vi "Dirac Integrand for Gated Decay.vi"(8 "Error In":errorcluster, 11 "data":variant) -> (0 "Error Out":errorcluster, 3 "F(X)":dbl)   [LabVIEW 2021, in "Phasor.lvlib"]
doc: "This template is the starting point for creating a function that is the integrand evaluation to be passed to the Quadrature.vi."
uses:
  Phasor.lvlib
  Phasor Gate & Decay Parameters.ctl
  Phasor Gate Type.ctl
  Phasor IRF Model.ctl
  Graphs/XY Graph/XY Graph Plot Data.ctl
  34e4ec69-d111-4f4b-ac3e-acf46f95d7c0.vi
  <vilib>/Utility/error.llb/Error Cluster From Error Code.vi
  Math/Math.lvlib
  Graphs/XY Graph/XY Graph Add-Ons.lvlib
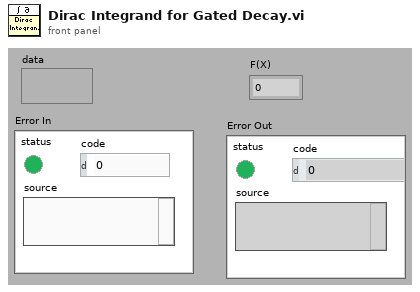
[diagram p1: front panel]
types:
  T1 = typedef "Phasor.lvlib/Phasor Gate & Decay Parameters.ctl" = cluster{"W":dbl, "T":dbl, "tau":dbl, "t_0":dbl, "Gate Type":T2, "t_i":dbl, "sR":dbl, "sF":dbl, "s":dbl, "Reversed Sawtooth":bool, "IRF Model":T3, "IRF Parameter 1":dbl, "User-defined Gate":T4, "Type of User-defined Function":enum32{"Gate", "IRF"}, "A":dbl}
  T2 = typedef "Phasor.lvlib/Phasor Gate Type.ctl" = enum16{"Square", "Finite Edge Square", "Finite Edge, Tilted Top Square", "Triangle", "Sawtooth", "User-defined"}
  T3 = typedef "Phasor.lvlib/Phasor IRF Model.ctl" = enum16{"Dirac", "Exponential"}
  T4 = typedef "XY Graph Add-Ons.lvlib/XY Graph Plot Data.ctl" = cluster{"X Array":dbl[], "Y Array":dbl[]}
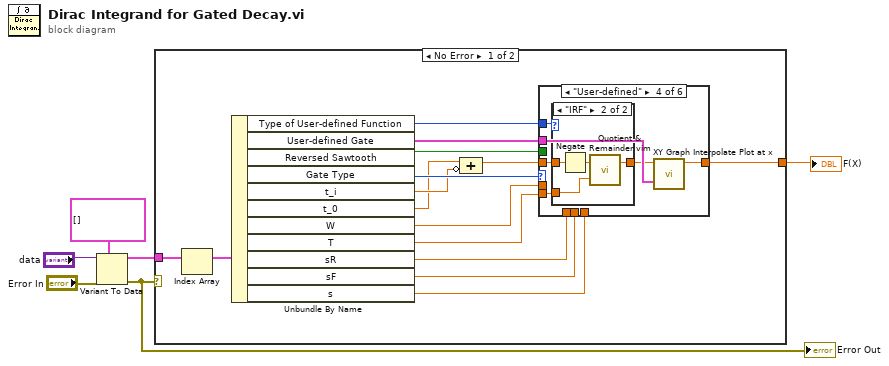
[diagram p0: block diagram]
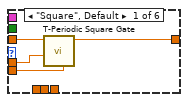
[diagram p2: hidden frame]
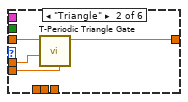
[diagram p3: hidden frame]
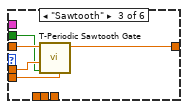
[diagram p4: hidden frame]
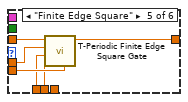
[diagram p6: hidden frame]
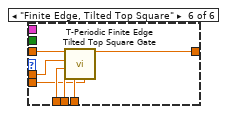
[diagram p7: hidden frame]
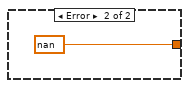
[diagram p8: hidden frame]
diagram:
  n1 = Variant To Data(error in="Error In", type=T1[] [] ("Array"), Variant="data") -> (data=w4:T1[], error out=w1:errorcluster)
  "Error Out" <- w1
  n2 = case shown="No Error" w1 {
    tunnel: w4 -> [w11 _]
    tunnel: [w8 nan ("Finite Edge Square(t)")] -> w3
    frame No Error {
      n3 = Index Array(array=w11) -> (element=w7:T1)  [unwired: 1 in]
      n4 = Unbundle By Name(w7) -> ("Type of User-defined Function"=w10:enum32{"Gate", "IRF"}, "User-defined Gate"=w12:T4, "Reversed Sawtooth"=w13:bool, "Gate Type"=w20:T2, "t_i"=w19:dbl, "t_0"=w9:dbl, "W"=w17:dbl, "T"=w21:dbl, "sR"=w16:dbl, "sF"=w15:dbl, "s"=w14:dbl)
      n5 = Compound Arithmetic op=ADD(w9, invert w19) -> (w18:dbl)
      n6 = case shown="\"User-defined\"" w20 {
        tunnel: w17 -> [w24 w29 w33 _ w49 w56]
        tunnel: w18 -> [w25 w28 w34 w40 w51 w58]
        tunnel: [w23 w27 w32 w39 w50 w57] -> w8
        tunnel: w16 -> [_ _ _ _ w47 w55]
        tunnel: w15 -> [_ _ _ _ w46 w54]
        tunnel: w14 -> [_ _ _ _ _ w53]
        tunnel: w13 -> [_ _ w31 _ _ _]
        tunnel: w12 -> [_ _ _ w38 _ _]
        tunnel: w21 -> [w22 w26 w30 w37 w48 w52]
        tunnel: w10 -> [_ _ _ w35 _ _]
        frame "Square", Default {
          n7 = call "T-Periodic Square Gate.vi"("Period T"=w22, "W"=w24, "t"=w25) -> ("Square(t)"=w23:dbl)  [unwired: 8 in]
        }
        frame "Triangle" {
          n8 = call "T-Periodic Triangle Gate.vi"("Period T"=w26, "W"=w29, "t"=w28) -> ("Triangle(t)"=w27:dbl)  [unwired: 8 in]
        }
        frame "Sawtooth" {
          n9 = call "T-Periodic Sawtooth Gate.vi"("Period T"=w30, "Reversed?"=w31, "W"=w33, "t"=w34) -> ("Sawtooth(t)"=w32:dbl)  [unwired: 7 in]
        }
        frame "User-defined" {
          n10 = case shown="\"IRF\"" w35 {
            tunnel: w40 -> [w41 w45]
            tunnel: w37 -> [_ w42]
            tunnel: [w41 w43] -> w36
            frame "Gate", Default {
            }
            frame "IRF" {
              n11 = Negate(x=w45) -> (-x=w44:dbl)
              n12 = call "Quotient & Remainder.vim"("y"=w42, "x"=w44) -> ("x - E(x/y)y"=w43:dbl)  [unwired: 1 out]
            }
          }
          n13 = call "XY Graph Interpolate Plot at x.vi"("XY Plot"=w38, "t"=w36) -> ("XY Plot(t)"=w39:dbl)  [unwired: 8 in, 1 out]
        }
        frame "Finite Edge Square" {
          n14 = call "T-Periodic Finite Edge Square Gate.vi"("Period T"=w48, "s_F"=w46, "s_R"=w47, "W"=w49, "t"=w51) -> ("Finite Edge Square(t)"=w50:dbl)  [unwired: 6 in]
        }
        frame "Finite Edge, Tilted Top Square" {
          n15 = call "T-Periodic Finite Edge Tilted Top Square Gate.vi"("Period T"=w52, "slope"=w53, "s_F"=w54, "s_R"=w55, "W"=w56, "t"=w58) -> ("Finite Edge Square(t)"=w57:dbl)  [unwired: 5 in]
        }
      }
    }
    frame Error {
    }
  }
  "F(X)" <- w3
